vi "Untitled 1.vi"() -> ()   [LabVIEW 2024]
uses:
  <vilib>/DAQmx/miscellaneous.llb/DAQmx Fill In Error Info.vi
  <vilib>/DAQmx/read.llb/DAQmx Read (Analog DBL 1Chan 1Samp).vi
panel:
  out "Numeric":dbl
  in  "stop":bool
  out "Waveform Chart":dbl(graph)
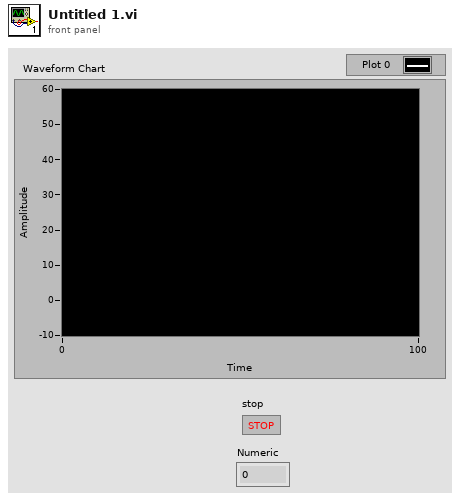
[diagram p1: front panel]
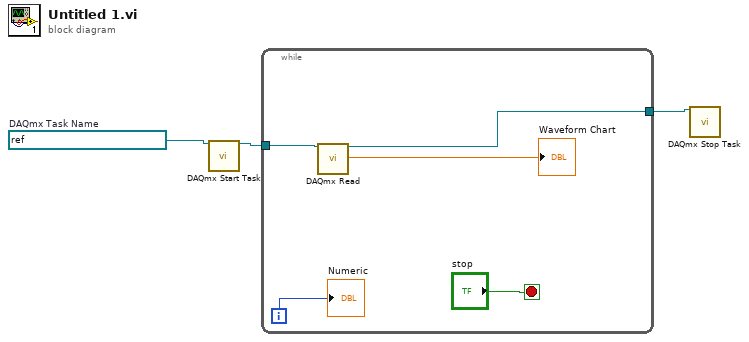
[diagram p0: block diagram]
diagram:
  w3 = refnum<k21> "VoltageSimulated"  # DAQmx Task Name
  n1 = call <vilib>:"DAQmx Start Task.vi"("task/channels in"=w3) -> ("task out"=w2:refnum<k21>)  [unwired: 13 in, 1 out]
  n2 = while {
    tunnel: w2 -> [w8]
    tunnel: [w6] -> w1
    i -> [w4]
    stop <- "stop" stop-if-true
    n3 = call-poly <vilib>:"DAQmx Read.vi"("task/channels in"=w8) -> ("task out"=w6:refnum<k21>, "data"=→"Waveform Chart":dbl)  [unwired: 12 in, 1 out]
    "Numeric" <- w4
  }
  n4 = call <vilib>:"DAQmx Stop Task.vi"("task/channels in"=w1) -> ()  [unwired: 13 in, 2 out]
